vi "ParseCalibData.vi"(8 "error in (no error)":errorcluster, 10 "Calib Registers":u8[](array[numeric]), 11 "BME680 in":refnum<class "BME680.lvclass">) -> (0 "error out":errorcluster, 3 "BME680 out":refnum<class "BME680.lvclass">)   [LabVIEW 2022 SP3, in "BME680.lvlib" / "BME680.lvclass"]
uses:
  BME680.lvclass
  BME680.lvclass/BME680.ctl
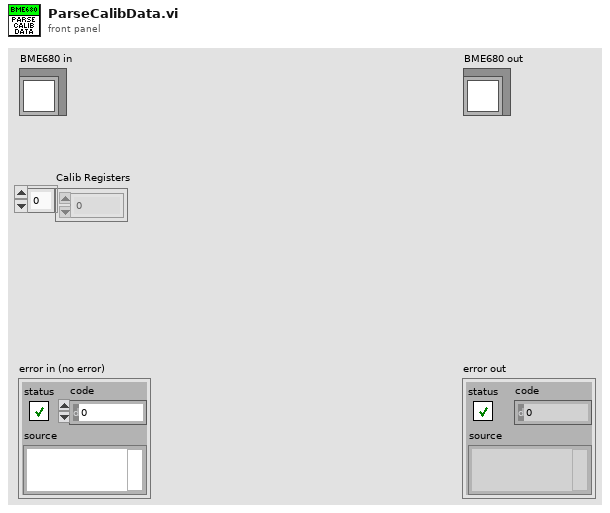
[diagram p1: front panel]
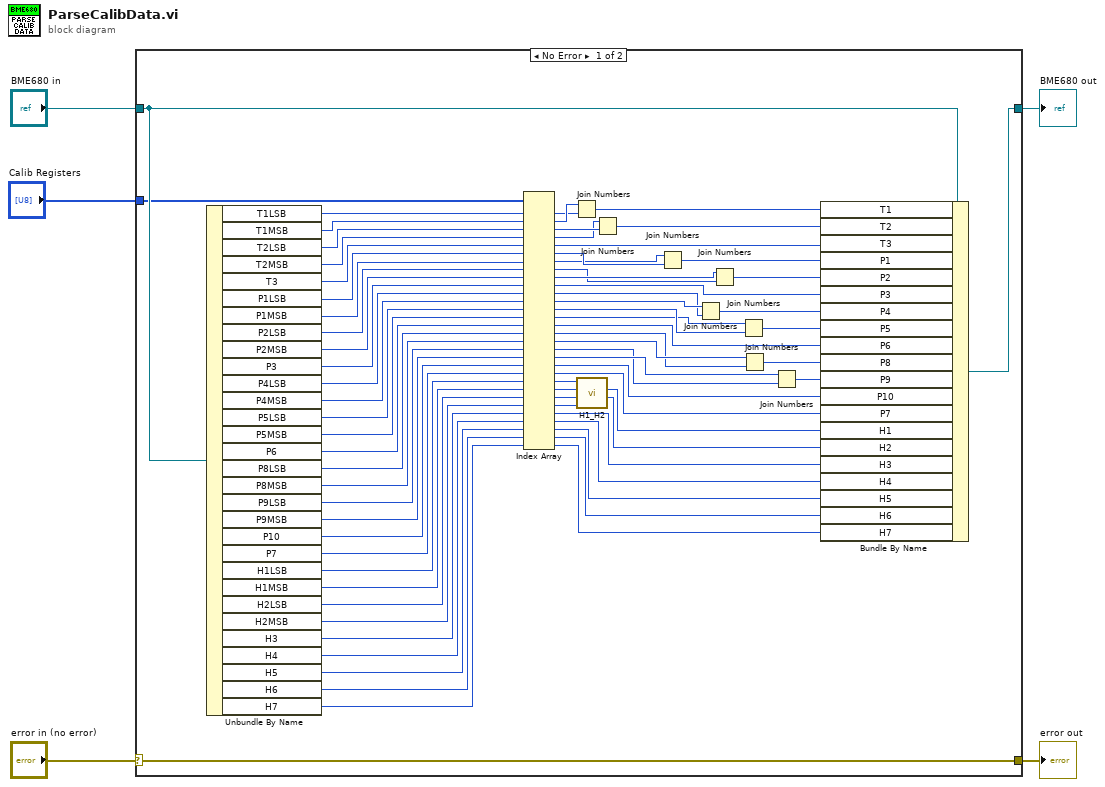
[diagram p0: block diagram]
diagram:
  n1 = case shown="No Error" "error in (no error)" {
    selector: "error in (no error)" -> [w79 w81]
    tunnel: [w79 w81] -> w4
    tunnel: [w77 w80] -> w2
    tunnel: "BME680 in" -> [w78 w80]
    tunnel: "Calib Registers" -> [w76 _]
    frame No Error {
      n2 = Unbundle By Name(w78) -> ("T1LSB"=w75:u8, "T1MSB"=w74:u8, "T2LSB"=w73:u8, "T2MSB"=w72:u8, "T3"=w71:u8, "P1LSB"=w70:u8, "P1MSB"=w69:u8, "P2LSB"=w68:u8, "P2MSB"=w67:u8, "P3"=w66:u8, "P4LSB"=w65:u8, "P4MSB"=w64:u8, "P5LSB"=w63:u8, "P5MSB"=w62:u8, "P6"=w61:u8, "P8LSB"=w60:u8, "P8MSB"=w59:u8, "P9LSB"=w58:u8, "P9MSB"=w57:u8, "P10"=w56:u8, "P7"=w55:u8, "H1LSB"=w54:u8, "H1MSB"=w53:u8, "H2LSB"=w52:u8, "H2MSB"=w51:u8, "H3"=w50:u8, "H4"=w49:u8, "H5"=w48:u8, "H6"=w47:u8, "H7"=w46:u8)
      n3 = Index Array(array=w76, index #1=w75, index #2=w74, index #3=w73, index #4=w72, index #5=w71, index #6=w70, index #7=w69, index #8=w68, index #9=w67, index #10=w66, index #11=w65, index #12=w64, index #13=w63, index #14=w62, index #15=w61, index #16=w60, index #17=w59, index #18=w58, index #19=w57, index #20=w56, index #21=w55, index #22=w54, index #23=w53, index #24=w52, index #25=w51, index #26=w50, index #27=w49, index #28=w48, index #29=w47, index #30=w46) -> (element #1=w44:u8, element #2=w45:u8, element #3=w42:u8, element #4=w41:u8, element #5=w39:u8, element #6=w38:u8, element #7=w37:u8, element #8=w34:u8, element #9=w35:u8, element #10=w32:u8, element #11=w30:u8, element #12=w31:u8, element #13=w28:u8, element #14=w22:u8, element #15=w21:u8, element #16=w8:u8, element #17=w9:u8, element #18=w6:u8, element #19=w7:u8, element #20=w10:u8, element #21=w11:u8, element #22=w12:u8, element #23=w13:u8, element #24=w14:u8, element #25=w15:u8, element #26=w16:u8, element #27=w17:u8, element #28=w18:u8, element #29=w19:u8, element #30=w20:u8)
      n4 = Join Numbers(hi=w45, lo=w44) -> ((hi.lo)=w43:u16)
      n5 = call "H1_H2.vi"("H2 MSB"=w15, "H2 LSB"=w14, "H1 MSB"=w13, "H1 LSB"=w12) -> ("H2"=w23:u16, "H1"=w24:u16)  [unwired: 6 in]
      n6 = Join Numbers(hi=w41, lo=w42) -> ((hi.lo)=w40:u16)
      n7 = Join Numbers(hi=w37, lo=w38) -> ((hi.lo)=w36:u16)
      n8 = Join Numbers(hi=w31, lo=w30) -> ((hi.lo)=w29:u16)
      n9 = Join Numbers(hi=w35, lo=w34) -> ((hi.lo)=w33:u16)
      n10 = Join Numbers(hi=w22, lo=w28) -> ((hi.lo)=w27:u16)
      n11 = Join Numbers(hi=w9, lo=w8) -> ((hi.lo)=w26:u16)
      n12 = Join Numbers(hi=w7, lo=w6) -> ((hi.lo)=w25:u16)
      n13 = Bundle By Name(cluster=w78, "T1"=w43, "T2"=w40, "T3"=w39, "P1"=w36, "P2"=w33, "P3"=w32, "P4"=w29, "P5"=w27, "P6"=w21, "P8"=w26, "P9"=w25, "P10"=w10, "P7"=w11, "H1"=w24, "H2"=w23, "H3"=w16, "H4"=w17, "H5"=w18, "H6"=w19, "H7"=w20) -> (w77:refnum<class "BME680.lvclass">)
    }
    frame Error {
    }
  }
  "error out" <- w4
  "BME680 out" <- w2
